vi "DOM document.vi"() -> ()   [LabVIEW 2024]
panel:
  in  "DOM document out 2":refnum<k20>
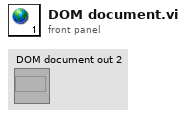
[diagram p1: front panel]
diagram:
